vi "Fetch Sensor Profile.vi"(8 "error in (no error)":errorcluster, 10 "SQL Query":string, 11 "Refnum in":T4) -> (0 "error out":errorcluster, 2 "Sensor CoreData Cluster":T1, 3 "Refnum out":T4)   [LabVIEW 2026, in "Database.lvlib"]
uses:
  Database.lvlib
  <vilib>/addons/database/Connection.llb/Conn ObjectReference.ctl
  controls/Messaging Payloads/Sensor CoreData Cluster.ctl
  controls/UI/Units Enum.ctl
  controls/UI/Signal Enum.ctl
  <vilib>/addons/database/Connection.llb/Conn Execute.vi
  <vilib>/addons/database/Recordset.llb/Rec Fetch String Data (R).vi
  <vilib>/addons/database/Recordset.llb/Rec Fetch Double Data (R).vi
  <vilib>/addons/database/Recordset.llb/Rec Fetch Integer Data (R).vi
  <vilib>/addons/database/Recordset.llb/Rec Destroy - Connection.vi
  <vilib>/addons/database/NI_Database_API.lvlib
  Settings/Settings.lvlib
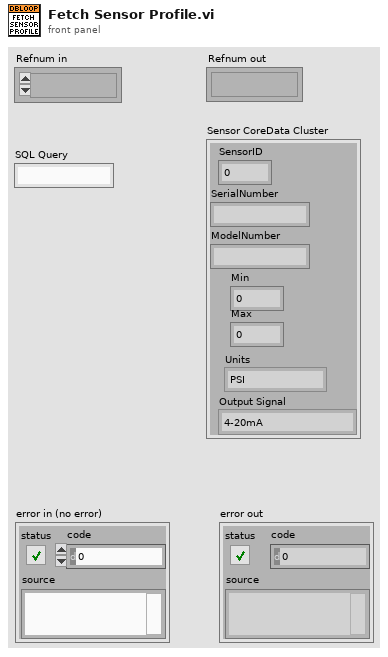
[diagram p1: front panel]
types:
  T1 = typedef "Settings.lvlib/Sensor CoreData Cluster.ctl" = cluster{"SensorID":i32, "SerialNumber":string, "ModelNumber":string, "Min":dbl, "Max":dbl, "Units":T2, "Output Signal":T3}
  T2 = typedef "Units Enum.ctl" = enum16{"PSI", "Deg C", "kPa", "GPM"}
  T3 = typedef "Signal Enum.ctl" = enum16{"4-20mA", "0-10V", "Thermocouple Type K"}
  T4 = typedef "NI_Database_API.lvlib/Conn ObjectReference.ctl" = refnum<k1>
  T5 = typedef "NI_Database_API.lvlib/Rec ObjectReference.ctl" = refnum<k1>
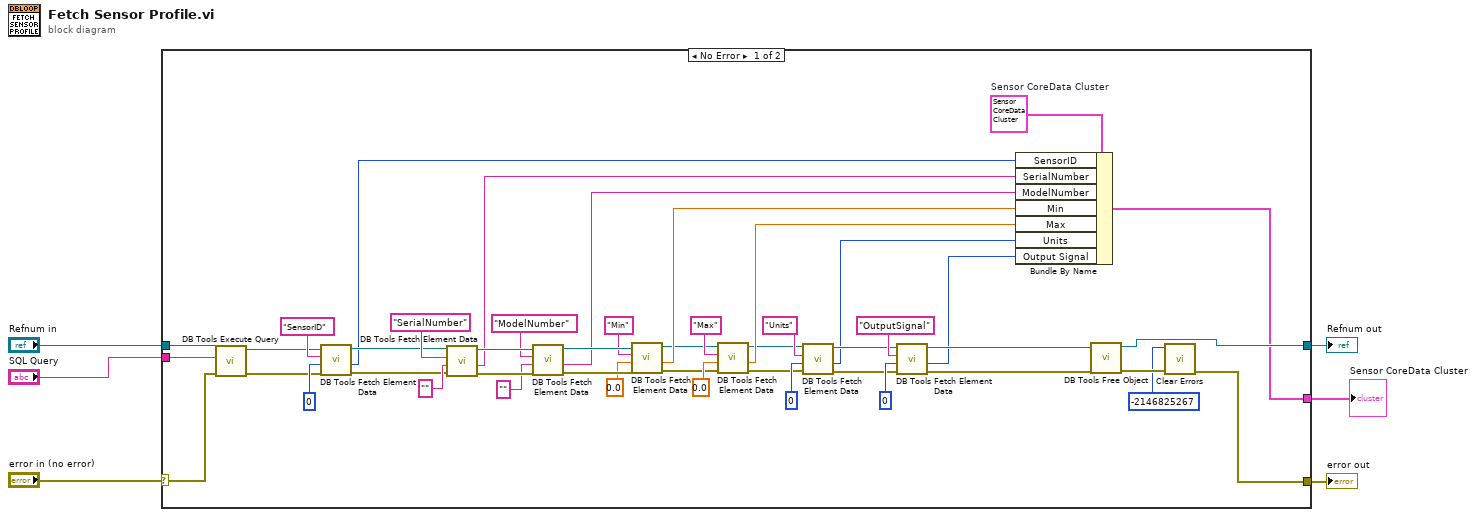
[diagram p0: block diagram]
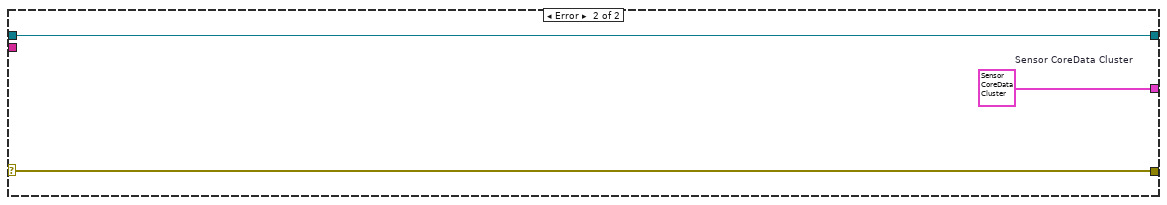
[diagram p2: hidden frame]
diagram:
  n1 = case shown="No Error" "error in (no error)" {
    selector: "error in (no error)" -> [w37 w55]
    tunnel: [w52 w54] -> w6
    tunnel: [w51 w55] -> w5
    tunnel: "SQL Query" -> [w48 _]
    tunnel: "Refnum in" -> [w47 w54]
    tunnel: [w14 w53] -> w1
    frame No Error {
      w15 = T1 {"SensorID"=0, "SerialNumber"="", "ModelNumber"="", "Min"=0.0, "Max"=0.0, "Units"=enum."PSI", "Output Signal"=enum."4-20mA"}  # Sensor CoreData Cluster
      n2 = call-poly <vilib>:"DB Tools Execute Query.vi"("error in (no error)"=w37, "SQL query"=w48, "connection reference"=w47) -> ("error out"=w11:errorcluster, "recordset reference"=w9:T5)  [unwired: 5 in]
      n3 = call-poly <vilib>:"DB Tools Fetch Element Data.vi"("error in (no error)"=w11, "type"=0, "column index"="SensorID", "recordset reference"=w9) -> ("error out"=w10:errorcluster, "data"=w7:i32, "recordset reference out"=w8:T5)  [unwired: 3 in]
      n4 = call-poly <vilib>:"DB Tools Fetch Element Data.vi"("error in (no error)"=w10, "type"="", "column index"="SerialNumber", "recordset reference"=w8) -> ("error out"=w41:errorcluster, "data"=w16:string, "recordset reference out"=w40:T5)  [unwired: 3 in]
      n5 = call-poly <vilib>:"DB Tools Fetch Element Data.vi"("error in (no error)"=w41, "type"="", "column index"="ModelNumber", "recordset reference"=w40) -> ("error out"=w44:errorcluster, "data"=w17:string, "recordset reference out"=w45:T5)  [unwired: 3 in]
      n6 = call-poly <vilib>:"DB Tools Fetch Element Data.vi"("error in (no error)"=w44, "type"=0.0, "column index"="Min", "recordset reference"=w45) -> ("error out"=w27:errorcluster, "data"=w46:dbl, "recordset reference out"=w28:T5)  [unwired: 3 in]
      n7 = call-poly <vilib>:"DB Tools Fetch Element Data.vi"("error in (no error)"=w27, "type"=0.0, "column index"="Max", "recordset reference"=w28) -> ("error out"=w23:errorcluster, "data"=w26:dbl, "recordset reference out"=w21:T5)  [unwired: 3 in]
      n8 = call-poly <vilib>:"DB Tools Fetch Element Data.vi"("error in (no error)"=w23, "type"=0, "column index"="Units", "recordset reference"=w21) -> ("error out"=w22:errorcluster, "data"=w19:i32, "recordset reference out"=w20:T5)  [unwired: 3 in]
      n9 = call-poly <vilib>:"DB Tools Fetch Element Data.vi"("error in (no error)"=w22, "type"=0, "column index"="OutputSignal", "recordset reference"=w20) -> ("error out"=w35:errorcluster, "data"=w18:i32, "recordset reference out"=w36:T5)  [unwired: 3 in]
      n10 = Bundle By Name(cluster=w15, "SensorID"=w7, "SerialNumber"=w16, "ModelNumber"=w17, "Min"=w46, "Max"=w26, "Units"=w19, "Output Signal"=w18) -> (w14:T1)
      n11 = call-poly <vilib>:"DB Tools Free Object.vi"("error in (no error)"=w35, "recordset reference"=w36) -> ("error out"=w50:errorcluster, "connection reference"=w52:T4)  [unwired: 8 in]
      n12 = call <vilib>:"Clear Errors.vi"("error in (no error)"=w50, "specific error code to clear (0: all)"=-2146825267) -> ("error out"=w51:errorcluster)  [unwired: 4 in, 1 out]
    }
    frame Error {
      w53 = T1 {"SensorID"=0, "SerialNumber"="", "ModelNumber"="", "Min"=0.0, "Max"=0.0, "Units"=enum."PSI", "Output Signal"=enum."4-20mA"}  # Sensor CoreData Cluster
    }
  }
  "Refnum out" <- w6
  "error out" <- w5
  "Sensor CoreData Cluster" <- w1
